vi "Write Data.vi"(8 "error in (no error)":errorcluster, 9 "Publication Time":timestamp, 10 "Value":variant, 11 "ControlCaptionBinding in":refnum<class "ControlCaptionBinding.lvclass">) -> (0 "error out":errorcluster, 3 "ControlCaptionBinding out":refnum<class "ControlCaptionBinding.lvclass">)   [LabVIEW 2017, in "Transport.lvlib" / "ControlCaptionBinding.lvclass"]
doc: "<License>\nCopyright © 2017 Composed Systems, LLC | All rights reserved\nwww.composed.io\n\nAuthor: Ethan Stern <ethan.stern@composed.io>\n\nThis software is provided \"AS IS\" WITHOUT WARRANTIES, either express or implied, AND IS FOR EDUCATIONAL PURPOSES ONLY.\n</License>"
uses:
  ControlCaptionBinding.lvclass
  ControlCaptionBinding.lvclass/ControlCaptionBinding.ctl
  <vilib>/Utility/error.llb/Error Cluster From Error Code.vi
  <vilib>/ErrorRing/Error Ring.xnode
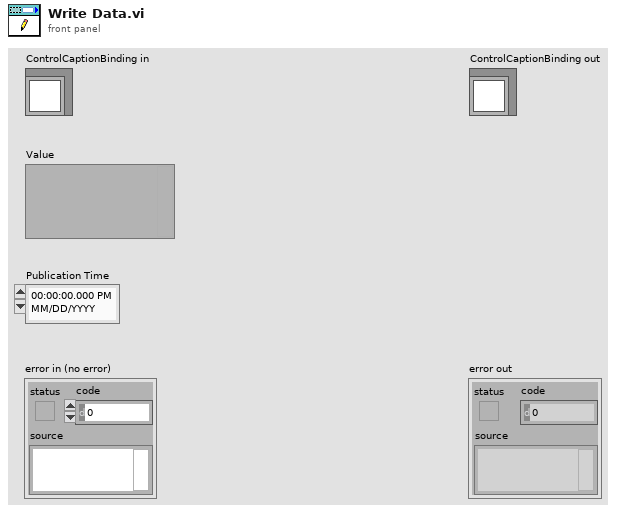
[diagram p1: front panel]
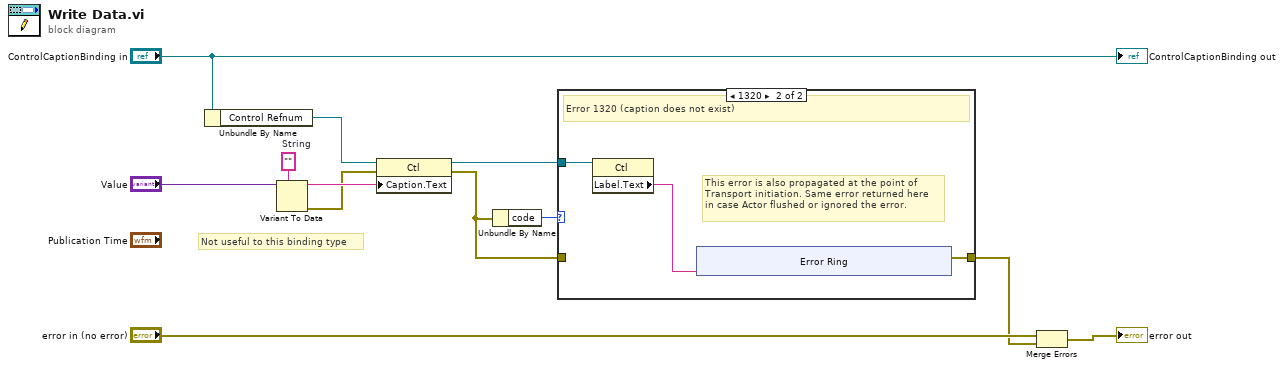
[diagram p0: block diagram]
diagram:
  w6 = ""  # String
  # "Not useful to this binding type"
  n1 = Unbundle By Name("ControlCaptionBinding in") -> ("Control Refnum"=w9:refnum<vi>)
  n2 = Variant To Data(type=w6, Variant="Value") -> (data=w8:string, error out=w5:errorcluster)  [unwired: 1 in]
  n3 = property class="Ctl"(reference=w9, error in=w5, "Caption.Text"=w8) -> (reference out=w4:refnum<vi>, error out=w2:errorcluster)
  n4 = Unbundle By Name(w2) -> ("code"=w1:i32)
  n5 = case shown="1320" w1 {
    tunnel: [w13 w16] -> w3
    tunnel: w4 -> [_ w15]
    tunnel: w2 -> [w13 _]
    frame 0, Default {
    }
    frame 1320 {
      # "This error is also propagated at the point of\nTransport initiation. Same error returned here\nin case Actor flushed or ignored the error."
      # "Error 1320 (caption does not exist)"
      n6 = property class="Ctl"(reference=w15) -> ("Label.Text"=w14:string)  [unwired: 1 in, 2 out]
      n7 = xnode "Error Ring"("parameter 0"=w14) -> ("error out"=w16:errorcluster)
    }
  }
  n8 = Merge Errors("error in (no error)", w3) -> (→"error out":errorcluster)
  "ControlCaptionBinding out" <- "ControlCaptionBinding in"
